vi "SUB_R_COM_FindString_timeout_new.vi"(4 "Find this String":string, 5 "Timeout Seccond":dbl, 6 "Begin time":dbl, 7 "duplicate VISA resource name 2":refnum<visa-resource-name>) -> (1 "Output String":string, 2 "spent seconds":dbl, 3 "Found String":bool)   [LabVIEW 2011]
panel:
  out "String":string
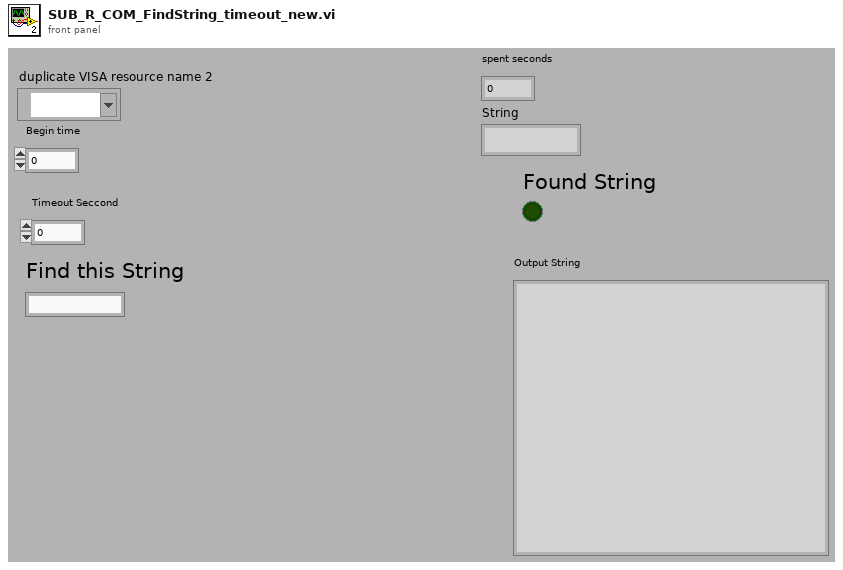
[diagram p1: front panel]
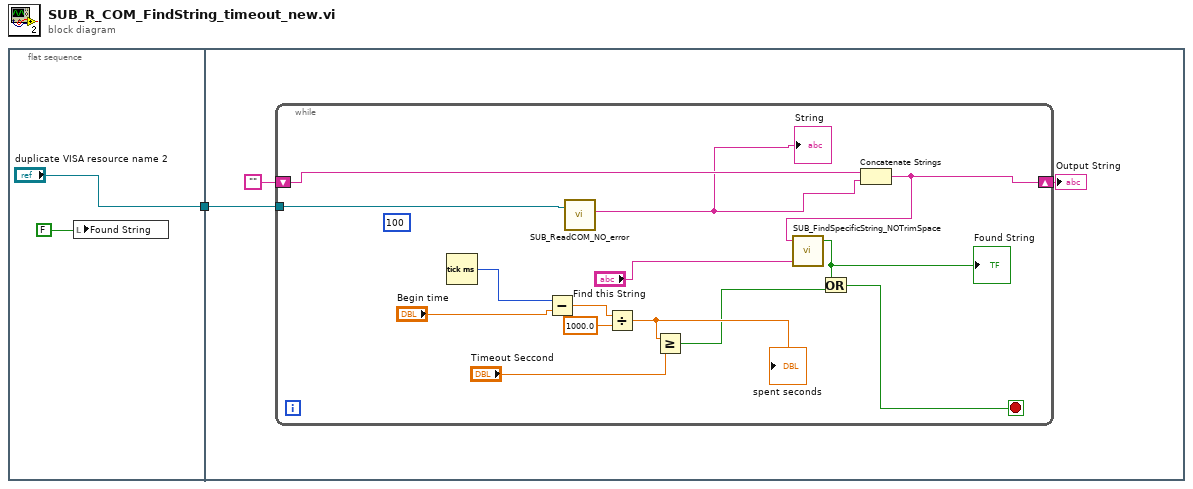
[diagram p0: block diagram]
diagram:
  n1 = flat-sequence {
    tunnel: ["duplicate VISA resource name 2"] -> w1
    tunnel: w1 -> [w4]
    frame #0 {
      n2 = local write "Found String"(FALSE) -> ()
    }
    frame #1 {
      n3 = while {
        shift-right: [w9] -> w5
        shift-left: "" -> [w12]
        tunnel: w4 -> [w8]
        stop <- w14 stop-if-true
        (unwired) 100 ("Numeric")
        n4 = Tick Count (ms)() -> (millisecond timer value=w11:u32)
        n5 = Subtract(x=w11, y="Begin time") -> (x-y=w20:dbl)
        n6 = call "SUB_ReadCOM_NO_error.vi"("VISA resource name"=w8) -> ("uart msg"=w7:string)  [unwired: 2 in, 2 out]
        "String" <- w7
        n7 = Divide(x=w20, y=1000.0) -> (x/y=w18:dbl)
        "spent seconds" <- w18
        n8 = Greater Or Equal?(x=w18, y="Timeout Seccond") -> (x >= y?=w15:bool)
        n9 = Concatenate Strings(w12, w7) -> (w9:string)
        n10 = call "SUB_FindSpecificString_NOTrimSpace.vi"("Find this String"="Find this String", "String data"=w9) -> ("Found"=w16:bool)  [unwired: 2 in, 1 out]
        "Found String" <- w16
        n11 = Or(x=w16, y=w15) -> (x .or. y?=w14:bool)
      }
      "Output String" <- w5
    }
  }
